vi "CSM DQMH-Style Template.vi"(7 "Name (\"\" to Use UUID)":string="CSM-Module") -> ()   [LabVIEW 2017]
doc: "------------- lvcsm -------------\n[CSMStates]\nItem 0 = \"Idle\"\nItem 1 = \"CSM Documentation\"\nItem 2 = \"VI Reference\"\nItem 3 = \"Error Handler\"\nItem 4 = \"Critical Error\"\nItem 5 = \"Target Timeout Error\"\nItem 6 = \"Target Error\"\nItem 7 = \"Async Response\"\nItem 8 = \"Response\"\nItem 9 = \"Async Message Posted\"\nItem 10 = \"Initialize Core Data\"\nItem 11 = \"Exit\"\nItem 12 = \"Data: Initialize\"\nItem 13 = \"Data: Update Indicators\"\nItem 14 = \"Data: Cleanup\"\nItem 15 = \"Macro: Initialize\"\nItem 16 = \"Macro: Exit\"\nItem 17 = \"API: API1\"\nItem 18 = \"API: API2\"\nItem 19 = \"Action: action1\"\nItem 20 = \"Action: action2\"\n\n[CSMStatus]\nItem 0 = \"Error Occurred@Error Handler\""
uses:
  user.lib/_NEVSTOP/Communicable State Machine(CSM)/AdvanceAPI/CSM - Revert Arguments-Safe String.vi
  user.lib/_NEVSTOP/Communicable State Machine(CSM)/AdvanceAPI/CSM - Break Down Multiple States String.vi
  user.lib/_NEVSTOP/Communicable State Machine(CSM)/AdvanceAPI/CSM - Compact Multiple States.vi
  user.lib/_NEVSTOP/Communicable State Machine(CSM)/AdvanceAPI/CSM - Make String Arguments Safe.vi
  user.lib/_NEVSTOP/Communicable State Machine(CSM)/AdvanceAPI/CSM - Keywords.vi
  user.lib/_NEVSTOP/Communicable State Machine(CSM)/_Shared/Trim Single-line Text.vi
  user.lib/_NEVSTOP/Communicable State Machine(CSM)/_Polymophic/CSM - Filter Duplicated Lines.vi
  user.lib/_NEVSTOP/Communicable State Machine(CSM)/Communicable State Machine.lvlib
panel:
  in  "Slide":dbl(slide) caption="Flood of Events:\n\nPanel/Pane Size Event\nSlide/Knob... User Event by dragging\nNumeric Control Value Change Event by Arraw Button" scale=0.0..10.0
  out "Error Occurred":errorcluster
  out "State History":string
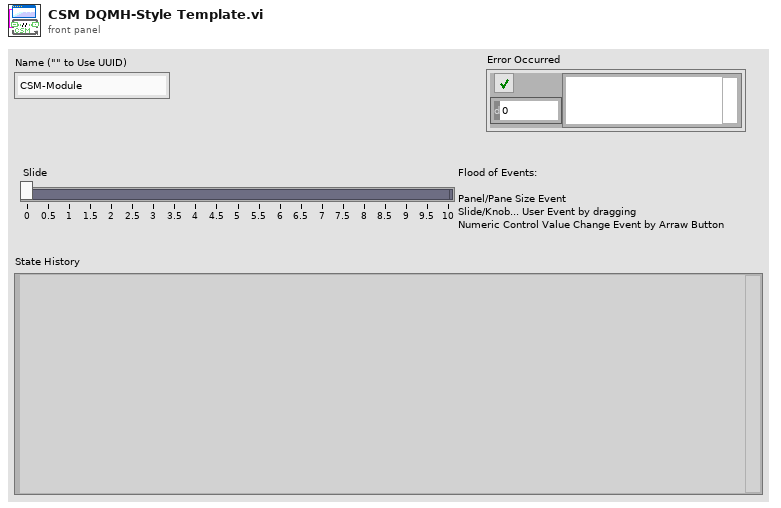
[diagram p1: front panel]
types:
  T1 = enum32{"Invalid", "Standard", "Closed", "Hidden", "Minimized", "Maximized"}
  T2 = enum32{"invalid app kind", "Development System", "Run Time System", "Student Edition", "Embedded LabVIEW", "Evaluation", "Custom"}
  T3 = typedef "Communicable State Machine.lvlib/_CSM_Response Source Message.ctl" = cluster{"‘State":string, "’Arguments":string, "’Error":errorcluster}
  T4 = cluster{"Current VI Reference":refnum<vi>, "Close Panel on Exit?":bool}
  T5 = cluster{"Core":cluster{"Current VI Reference":refnum<vi>, "Close Panel on Exit?":bool}, "Your Boolean data":bool, "Your string data":string}
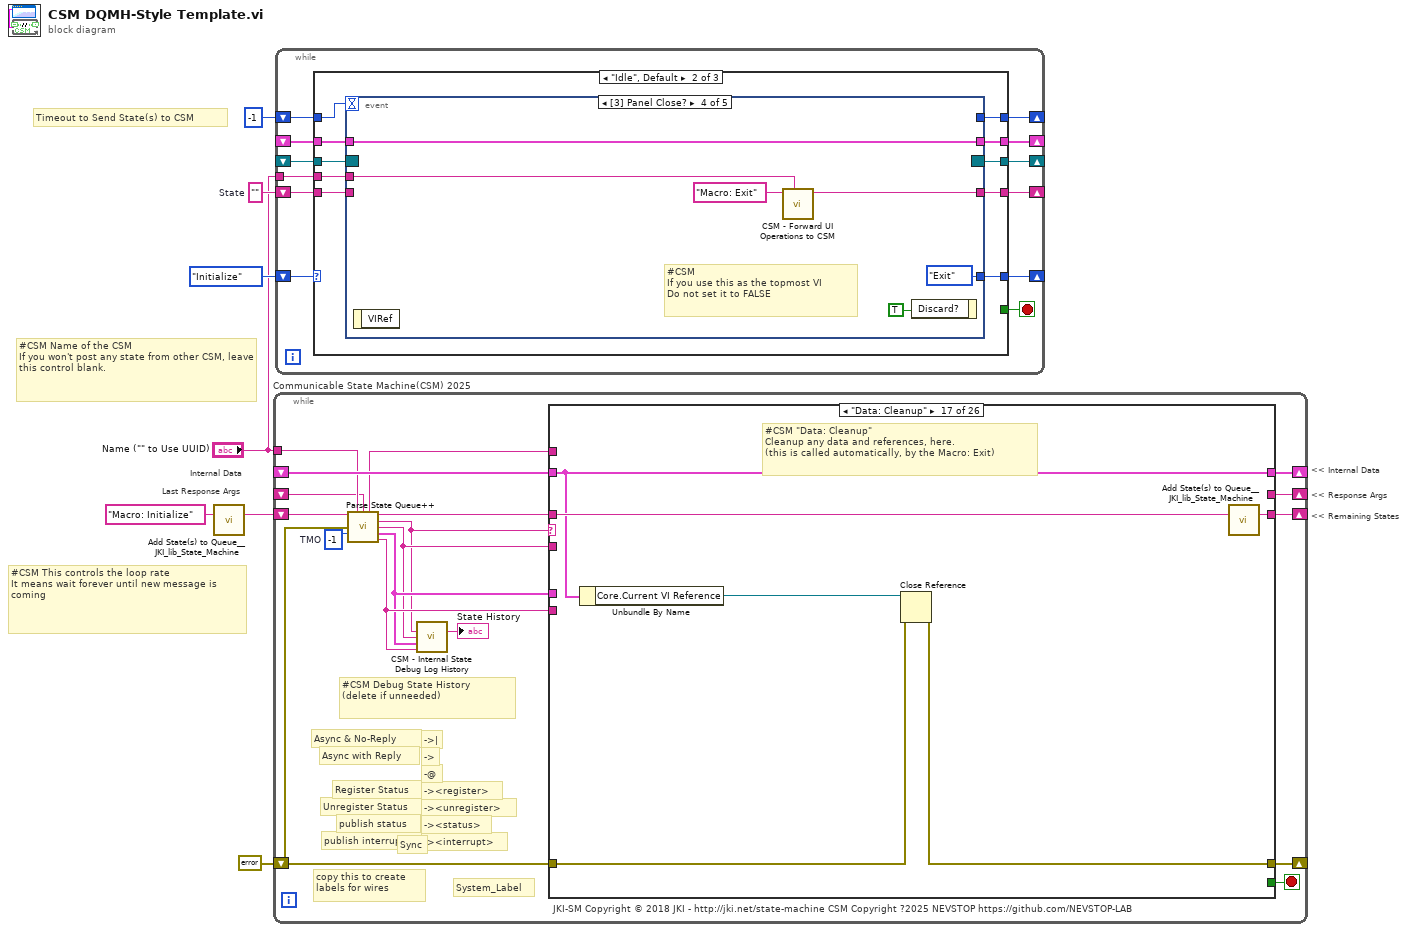
[diagram p0: block diagram]
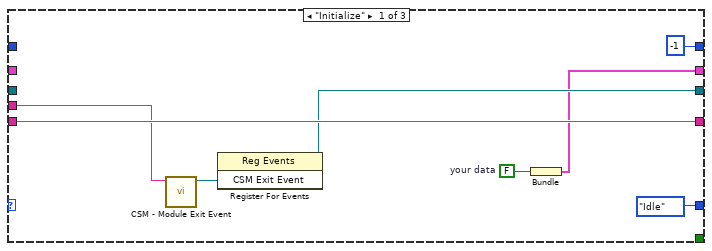
[diagram p2: hidden frame]
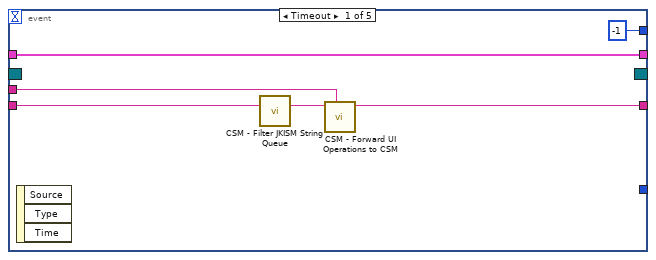
[diagram p3: hidden frame]
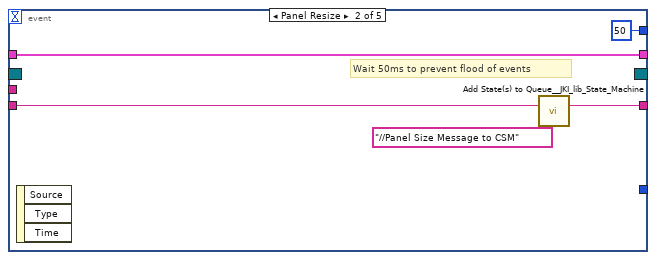
[diagram p4: hidden frame]
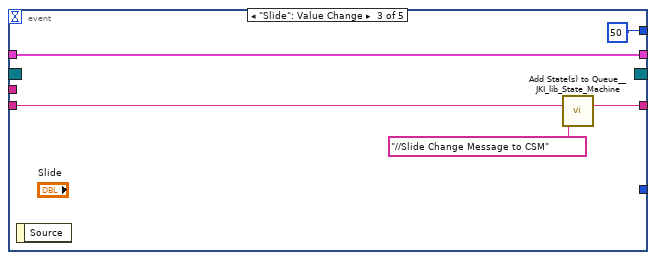
[diagram p5: hidden frame]
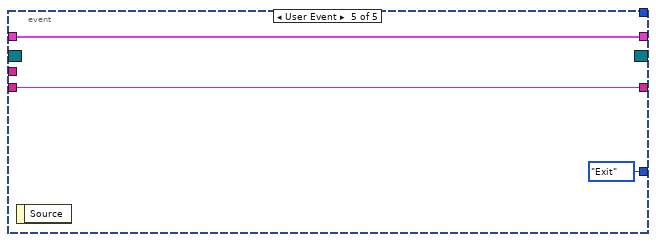
[diagram p6: hidden frame]
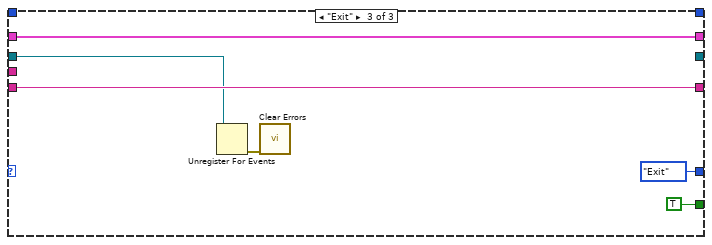
[diagram p7: hidden frame]
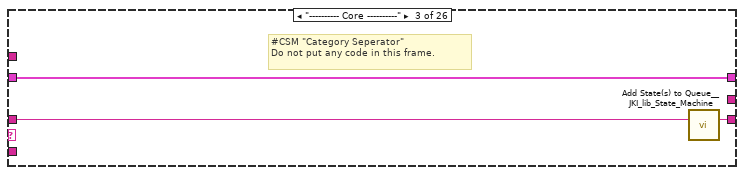
[diagram p10: hidden frame]
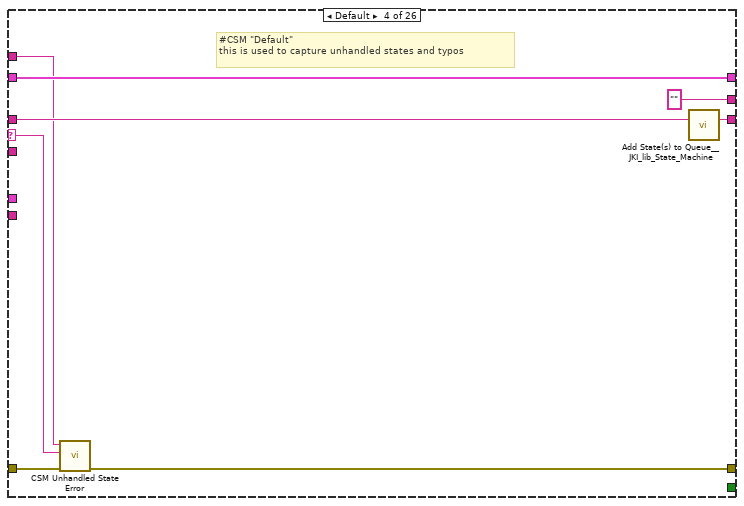
[diagram p11: hidden frame]
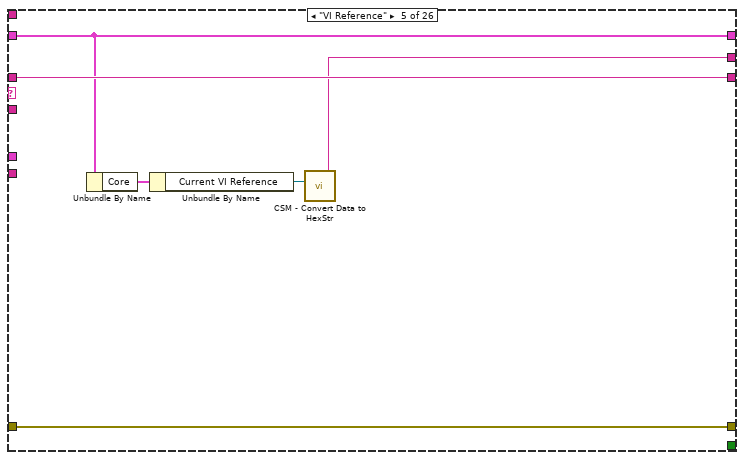
[diagram p12: hidden frame]
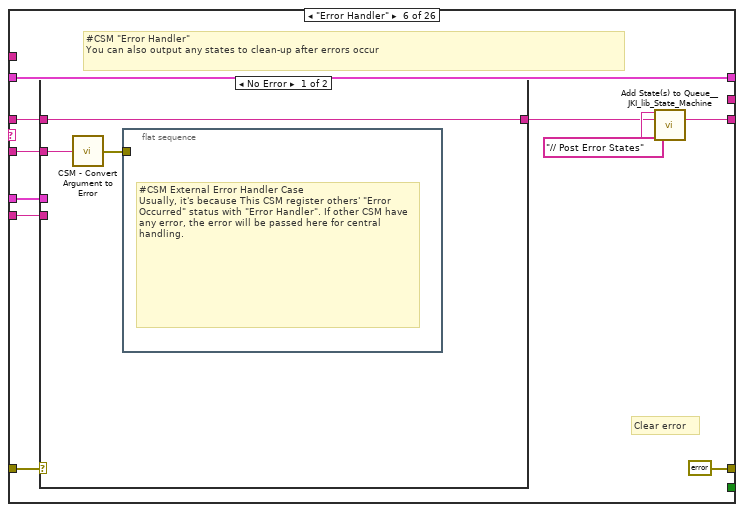
[diagram p13: hidden frame]
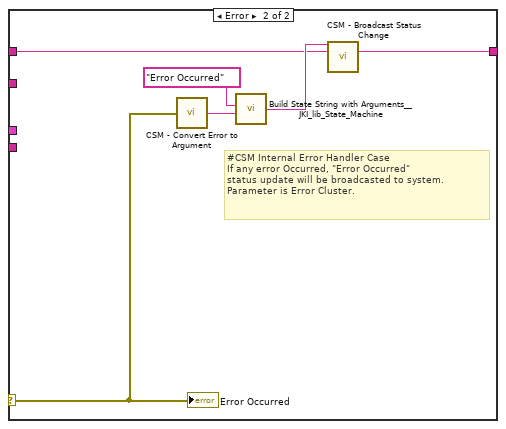
[diagram p14: hidden frame]
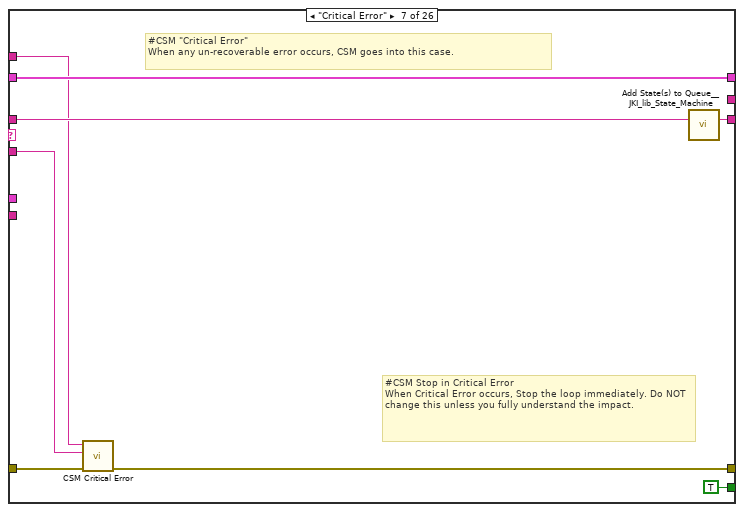
[diagram p15: hidden frame]
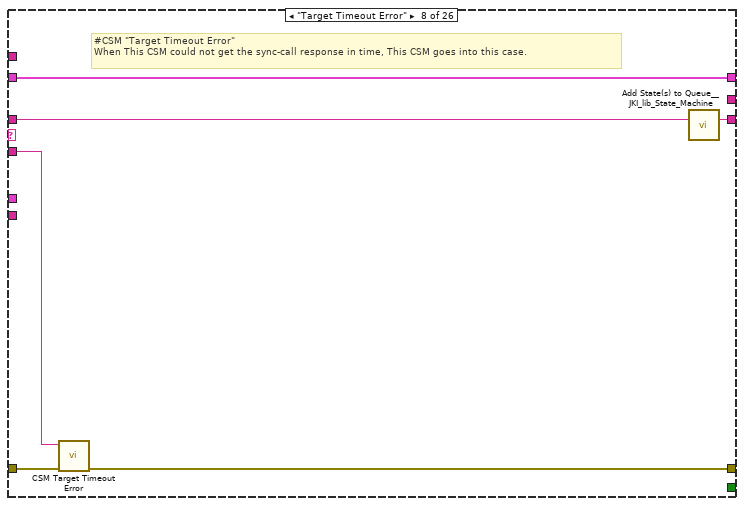
[diagram p16: hidden frame]
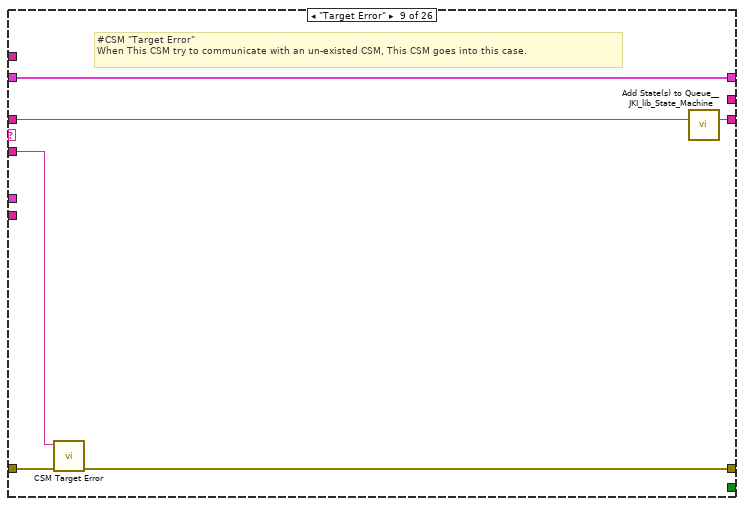
[diagram p17: hidden frame]
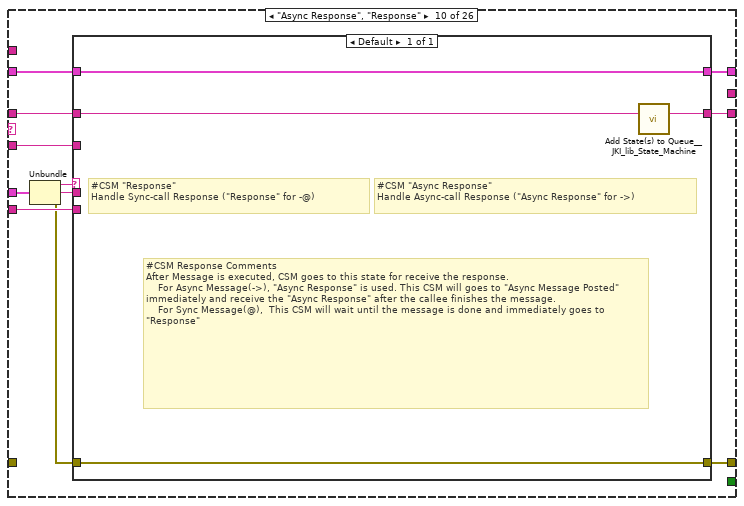
[diagram p18: hidden frame]
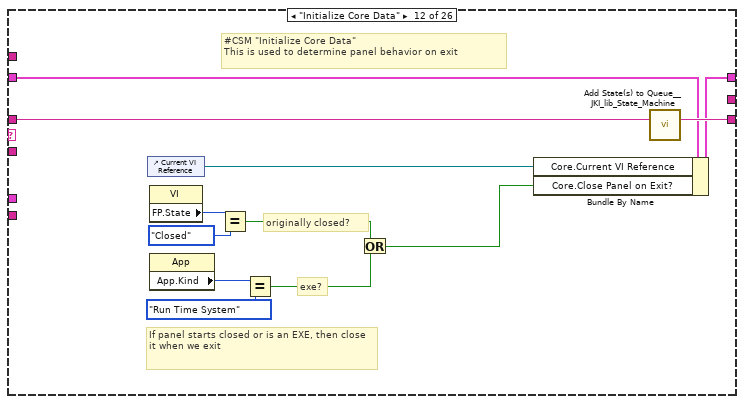
[diagram p20: hidden frame]
diagram:
  w3 = ""  # State
  # "Timeout to Send State(s) to CSM"
  # "Last Response Args"
  # "Internal Data"
  # "#CSM Name of the CSM\nIf you won't post any state from other CSM, leave this control blank."
  # "#CSM This controls the loop rate\nIt means wait forever until new message is coming"
  # "<< Internal Data"
  # "<< Response Args"
  # "<< Remaining States"
  n1 = call <vilib>:"Add State(s) to Queue__JKI_lib_State_Machine.vi"("State(s) in (\"\")"="Macro: Initialize" ("Init State(\"Macro: Initialize\")")) -> ("States Out"=w7:string)  [unwired: 14 in]
  n2 = while "Communicable State Machine(CSM) 2025" {
    shift-right: [w20] -> _
    shift-left: _ -> [w19]
    shift-right: [w23] -> _
    shift-left: errorcluster {"status"=FALSE, "code"=0, "source"=""} ("error out") -> [w9]
    shift-right: [w22] -> _
    shift-left: w7 -> [w24]
    tunnel: "Name (\"\" to Use UUID)" -> [w16]
    shift-right: [w17] -> _
    shift-left: _ -> [w11]
    stop <- w21 stop-if-true
    w18 = -1  # TMO
    # "#CSM Debug State History\n(delete if unneeded)"
    # "-><interrupt>"
    # "-><status>"
    # "-><unregister>"
    # "-><register>"
    # "-@"
    # "->"
    # "->|"
    # "publish interrupt"
    # "publish status"
    # "Unregister Status"
    # "Register Status"
    # "Sync"
    # "Async with Reply"
    # "Async & No-Reply"
    # "JKI-SM Copyright © 2018 JKI - http://jki.net/state-machine CSM Copyright ?2025 NEVSTOP https://github.com/NEVSTOP-LAB"
    # "copy this to create labels for wires"
    # "System_Label"
    n3 = call "Parse State Queue++.vi"("State Queue"=w24, "Name (\"\" to Use UUID)"=w16, "Response Arguments"=w11, "Previous Error"=w9, "Dequeue (1 ms)"=w18) -> ("Name Used"=w10:string, "Remaining States"=w25:string, "Current State"=w12:string, "Arguments"=w13:string, "Additional Information"=w14:T3, "Source CSM"=w15:string)  [unwired: 5 in]
    n4 = call "CSM - Internal State Debug Log History.vi"("State"=w12, "Arguments (\"\")"=w13, ">> Response Source Message >>"=w14, "Source (\"\")"=w15) -> ("Debug Log"=→"State History":string)  [unwired: 11 in]
    n5 = case shown="\"Data: Cleanup\"" w12 {
      selector: w12 -> [_ _ _ w36 _ _ _ _ _ _ _ _ _ _ _ _ _ _ _ _ _ _ _ _ _ _]
      tunnel: w25 -> [w26 w29 w32 w40 w45 w50 w73 w79 w85 w95 w102 w114 w118 w121 w127 w129 w135 w138 w142 w148 w150 w153 w157 w162 w165 w168]
      tunnel: w13 -> [_ _ _ _ _ w49 w69 w76 w82 w89 _ _ _ _ _ _ _ _ _ _ _ _ w155 _ _ _]
      tunnel: w19 -> [w27 w28 w30 w38 w44 w55 w71 w77 w83 w93 w101 w108 w116 w119 _ w128 w130 w136 w140 w146 w149 w152 w156 w160 w163 w166]
      tunnel: [_ _ _ w33 w46 errorcluster {"status"=FALSE, "code"=0, "source"=""} ("error out") w66 w74 w80 w96 _ _ _ _ _ _ w131 _ _ _ _ _ _ _ _ _] -> w23
      tunnel: w9 -> [_ _ _ w34 w46 w53 w67 w75 w81 _ _ _ _ _ _ _ w132 _ _ _ _ _ _ _ _ _]
      tunnel: [w26 w29 w31 w39 w45 w51 w72 w78 w84 w94 w102 w113 w117 w120 w126 w129 w134 w137 w141 w147 w150 w153 w157 w161 w164 w167] -> w22
      tunnel: [_ _ _ _ _ _ TRUE _ _ _ _ _ TRUE _ _ _ _ _ _ _ _ _ _ _ _ _] -> w21
      tunnel: [w27 w28 w30 w38 w44 w55 w71 w77 w83 w92 w101 w112 w116 w119 w125 w128 w130 w136 w140 w146 w149 w152 w156 w160 w163 w166] -> w20
      tunnel: w15 -> [_ _ _ _ _ w48 _ _ _ w90 _ _ _ _ _ _ _ _ _ _ _ _ _ _ _ _]
      tunnel: w14 -> [_ _ _ _ _ w47 _ _ _ w91 _ _ _ _ _ _ _ _ _ _ _ _ _ _ _ _]
      tunnel: [_ _ _ "" w41 _ _ _ _ _ _ _ _ _ _ _ _ _ _ _ _ "API1 Response" w154 _ _ _] -> w17
      tunnel: w10 -> [_ _ _ w35 _ _ w68 _ _ _ _ _ _ _ _ _ _ _ _ _ _ _ _ _ _ _]
      frame "", "Idle" {
        # "#CSM \"Idle/Event Handler\"\nexecutes when the state queue is empty"
      }
      frame "CSM Documentation" {
        # "#CSM State Syntax\n\n// Comment line, all text to the right of “//” will be ignored\n// Local Message Example\nDoSth: DoA >> Arguments\n\n// Sync Call Example\nAPI: xxxx >> Arguments -@ TargetModule\n\n// Async Call Example\nAPI: xxxx >> Arguments -> TargetModule\n\n// Async Call without Reply Example\nAPI: xxxx >> Arguments ->| TargetModule\n\n// Broadcast normal status:\nStatus >> StatusArguments  -><status>\n\n// Broadcast Interrupt status:\nInterrupt >> StatusArguments  -><interrupt>\n\n// Register Source Module's status to Handler Module\nStatus@Source Module >> Handler Module@Handler Module -><register>\n\n// Unegister Source Module's status\nStatus@Source Module >> Handler Module -><unregister>"
        # "#CSM README FIRST\n\nCommunicable State Machine(CSM) is a LabVIEW application framework that builds upon JKI State Machine(JKISM). It follows the pattern of JKISM and extends the keywords to describe message communication between modules, including concepts such as Sync-Message, Async-Message, Subscription/Unsubscription of status - essential elements for creating reusable code modules. For more information, please visit the CSM wiki: https://nevstop-lab.github.io/CSM-Wiki/\n\nFor instructions on JKI State Machine, visit: \n    http://jki.net/state-machine/\nFor information about CSM, visit: \n    https://github.com/NEVSTOP-LAB"
        # "#CSM \"Documentation\"\nCase for holding CSM Documenation"
      }
      frame "---------- Core ----------" {
        # "#CSM \"Category Seperator\"\nDo not put any code in this frame."
        n6 = call <vilib>:"Add State(s) to Queue__JKI_lib_State_Machine.vi"("State(s) in (\"\")"=w32) -> ("States Out"=w31:string)  [unwired: 14 in]
      }
      frame Default {
        # "#CSM \"Default\"\nthis is used to capture unhandled states and typos"
        n7 = call "CSM Unhandled State Error.vi"("error in (no error)"=w34, "Undefined State"=w36, "CSM Name"=w35) -> ("error out"=w33:errorcluster)  [unwired: 8 in]
        n8 = call <vilib>:"Add State(s) to Queue__JKI_lib_State_Machine.vi"("State(s) in (\"\")"=w40) -> ("States Out"=w39:string)  [unwired: 14 in]
      }
      frame "VI Reference" {
        n9 = Unbundle By Name(w44) -> ("Core"=w43:T4)
        n10 = Unbundle By Name(w43) -> ("Current VI Reference"=w42:refnum<vi>)
        n11 = call "CSM - Convert Data to HexStr.vi"("Variant"=w42) -> ("HEX String (0-9,A-F)"=w41:string)  [unwired: 8 in]
      }
      frame "Error Handler" {
        # "#CSM \"Error Handler\"\nYou can also output any states to clean-up after errors occur"
        # "Clear error"
        n12 = case shown="No Error" w53 {
          selector: w53 -> [_ w60]
          tunnel: [w59 w62] -> w52
          tunnel: w50 -> [w59 w61]
          tunnel: w49 -> [w58 _]
          tunnel: w48 -> [_ _]
          tunnel: w47 -> [_ _]
          frame No Error {
            n13 = call "CSM - Convert Argument to Error.vi"("Argument"=w58) -> ("Error"=w57:errorcluster)  [unwired: 4 in]
            n14 = flat-sequence {
              tunnel: w57 -> [_]
              frame #0 {
                # "#CSM External Error Handler Case\nUsually, it's because This CSM register others' \"Error Occurred\" status with \"Error Handler\". If other CSM have any error, the error will be passed here for central handling."
              }
            }
          }
          frame Error {
            # "#CSM Internal Error Handler Case \nIf any error Occurred, \"Error Occurred\" \nstatus update will be broadcasted to system.\nParameter is Error Cluster."
            n15 = call "CSM - Convert Error to Argument.vi"("Error"=w60) -> ("Argument"=w64:string)  [unwired: 4 in]
            n16 = call <vilib>:"Build State String with Arguments__JKI_lib_State_Machine.vi"("Arguments (\"\")"=w64, "State"="Error Occurred" ("Status with Arguments")) -> ("State with Arguments"=w63:string)  [unwired: 4 in]
            n17 = call "CSM - Broadcast Status Change.vi"("Status With Arguments"=w63, "State Queue"=w61) -> ("Remaining States"=w62:string)  [unwired: 13 in]
            "Error Occurred" <- w60
          }
        }
        n18 = call <vilib>:"Add State(s) to Queue__JKI_lib_State_Machine.vi"("State(s) in Front (\"\")"="// Post Error States", "State(s) in (\"\")"=w52) -> ("States Out"=w51:string)  [unwired: 13 in]
      }
      frame "Critical Error" {
        # "#CSM \"Critical Error\"\nWhen any un-recoverable error occurs, CSM goes into this case."
        # "#CSM Stop in Critical Error\nWhen Critical Error occurs, Stop the loop immediately. Do NOT change this unless you fully understand the impact."
        n19 = call "CSM Critical Error.vi"("error in (no error)"=w67, "Arugments (As Reason)"=w69, "CSM Name"=w68) -> ("error out"=w66:errorcluster)  [unwired: 8 in]
        n20 = call <vilib>:"Add State(s) to Queue__JKI_lib_State_Machine.vi"("State(s) in (\"\")"=w73) -> ("States Out"=w72:string)  [unwired: 14 in]
      }
      frame "Target Timeout Error" {
        # "#CSM \"Target Timeout Error\"\nWhen This CSM could not get the sync-call response in time, This CSM goes into this case."
        n21 = call "CSM Target Timeout Error.vi"("error in (no error)"=w75, "Arguments (As CSM Name)"=w76) -> ("error out"=w74:errorcluster)  [unwired: 9 in]
        n22 = call <vilib>:"Add State(s) to Queue__JKI_lib_State_Machine.vi"("State(s) in (\"\")"=w79) -> ("States Out"=w78:string)  [unwired: 14 in]
      }
      frame "Target Error" {
        # "#CSM \"Target Error\"\nWhen This CSM try to communicate with an un-existed CSM, This CSM goes into this case."
        n23 = call "CSM Target Error.vi"("error in (no error)"=w81, "Arguments (As CSM Name)"=w82) -> ("error out"=w80:errorcluster)  [unwired: 9 in]
        n24 = call <vilib>:"Add State(s) to Queue__JKI_lib_State_Machine.vi"("State(s) in (\"\")"=w85) -> ("States Out"=w84:string)  [unwired: 14 in]
      }
      frame "Async Response", "Response" {
        n25 = Unbundle(w91) -> ("‘State"=w88:string, "’Arguments"=w87:string, "’Error"=w86:errorcluster)
        n26 = case shown="Default" w88 {
          tunnel: [w97] -> w94
          tunnel: w95 -> [w98]
          tunnel: [w100] -> w92
          tunnel: w93 -> [w100]
          tunnel: [w99] -> w96
          tunnel: w86 -> [w99]
          tunnel: w90 -> [_]
          tunnel: w89 -> [_]
          tunnel: w87 -> [_]
          frame Default {
            # "#CSM \"Async Response\"\nHandle Async-call Response (\"Async Response\" for ->)"
            # "#CSM \"Response\"\nHandle Sync-call Response (\"Response\" for -@)"
            # "#CSM Response Comments\nAfter Message is executed, CSM goes to this state for receive the response.\n    For Async Message(->), \"Async Response\" is used. This CSM will goes to \"Async Message Posted\" immediately and receive the \"Async Response\" after the callee finishes the message.\n    For Sync Message(@),  This CSM will wait until the message is done and immediately goes to \"Response\""
            n27 = call <vilib>:"Add State(s) to Queue__JKI_lib_State_Machine.vi"("State(s) in (\"\")"=w98) -> ("States Out"=w97:string)  [unwired: 14 in]
          }
        }
      }
      frame "Async Message Posted" {
        # "#CSM \"Async Message Posted\"\nAfter Async Message is posted (-> or ->| ), CSM goes to this state for post-action.\nYou can use Argument - State to tell which Async Message is called."
      }
      frame "Initialize Core Data" {
        # "#CSM \"Initialize Core Data\"\nThis is used to determine panel behavior on exit"
        # "originally closed?"
        # "exe?"
        # "If panel starts closed or is an EXE, then close it when we exit"
        n28 = control-ref of="Current VI Reference"() -> (w106:refnum<vi>)
        n29 = property class="VI"() -> ("FP.State"=w105:T1)  [unwired: 2 in, 2 out]
        n30 = property class="App"() -> ("App.Kind"=w111:T2)  [unwired: 2 in, 2 out]
        n31 = Equal?(x=w105, y=T1."Closed" ("Front Panel Window:State")) -> (x = y?=w103:bool)
        n32 = Equal?(x=w111, y=T2."Run Time System" ("Application:Kind")) -> (x = y?=w109:bool)
        n33 = Or(x=w103, y=w109) -> (x .or. y?=w107:bool)
        n34 = Bundle By Name(cluster=w108, "Core.Current VI Reference"=w106, "Core.Close Panel on Exit?"=w107) -> (w112:T5)
        n35 = call <vilib>:"Add State(s) to Queue__JKI_lib_State_Machine.vi"("State(s) in (\"\")"=w114) -> ("States Out"=w113:string)  [unwired: 14 in]
      }
      frame "Exit" {
        # "#CSM \"Exit\"\nCase for exiting the loop. No errors that occur here will be handled."
        n36 = call <vilib>:"Add State(s) to Queue__JKI_lib_State_Machine.vi"("State(s) in (\"\")"=w118) -> ("States Out"=w117:string)  [unwired: 14 in]
      }
      frame "---------- Data ----------" {
        # "#CSM \"Category Seperator\"\nDo not put any code in this frame."
        n37 = call <vilib>:"Add State(s) to Queue__JKI_lib_State_Machine.vi"("State(s) in (\"\")"=w121) -> ("States Out"=w120:string)  [unwired: 14 in]
      }
      frame "Data: Initialize" {
        w122 = T4 {"Current VI Reference"=refnum, "Close Panel on Exit?"=FALSE}  # Core
        w124 = TRUE  # Your Boolean data
        w123 = ""  # Your string data
        # "#CSM \"Data: Initialize\"\nInitialize the shift-register data, here.\n(data names are defined by what you wire into the bundle function)"
        # "#CSM do not delete - used by framework"
        # "#CSM Expand Bundle to add new data elements to shift register data."
        # "#CSM Add new data here."
        # "#CSM Data names and types of shift register data are defined by this bundle."
        n38 = Bundle("Core"=w122, "Your Boolean data"=w124, "Your string data"=w123) -> (w125:T5)  [unwired: 1 in]
        n39 = call <vilib>:"Add State(s) to Queue__JKI_lib_State_Machine.vi"("State(s) in (\"\")"=w127) -> ("States Out"=w126:string)  [unwired: 14 in]
      }
      frame "Data: Update Indicators" {
      }
      frame "Data: Cleanup" {
        # "#CSM \"Data: Cleanup\"\nCleanup any data and references, here.\n(this is called automatically, by the Macro: Exit)"
        n40 = Unbundle By Name(w130) -> ("Core.Current VI Reference"=w133:refnum<vi>)
        n41 = Close Reference(reference=w133, error in (no error)=w132) -> (error out=w131:errorcluster)
        n42 = call <vilib>:"Add State(s) to Queue__JKI_lib_State_Machine.vi"("State(s) in (\"\")"=w135) -> ("States Out"=w134:string)  [unwired: 14 in]
      }
      frame "---------- Macro ----------" {
        # "#CSM \"Category Seperator\"\nDo not put any code in this frame."
        n43 = call <vilib>:"Add State(s) to Queue__JKI_lib_State_Machine.vi"("State(s) in (\"\")"=w138) -> ("States Out"=w137:string)  [unwired: 14 in]
      }
      frame "Macro: Initialize" {
        # "#CSM \"Macro: Initialize\"\nInitialization Macro (This is called once, when the VI starts)"
        n44 = call <vilib>:"Add State(s) to Queue__JKI_lib_State_Machine.vi"("State(s) in Front (\"\")"="Data: Initialize\nInitialize Core Data\nData: Update Indicators", "State(s) in (\"\")"=w142) -> ("States Out"=w141:string)  [unwired: 13 in]
      }
      frame "Macro: Exit" {
        # "#CSM \"Macro: Exit\"\nExit Macro (This is called once, when the VI exits)"
        n45 = call <vilib>:"Add State(s) to Queue__JKI_lib_State_Machine.vi"("State(s) in Front (\"\")"="//Exit Sub-Modules ", "State(s) at Back (\"\")"="Data: Cleanup\nExit") -> ("States Out"=w144:string)  [unwired: 13 in]
        n46 = call <vilib>:"Add State(s) to Queue__JKI_lib_State_Machine.vi"("State(s) in Front (\"\")"=w144, "State(s) in (\"\")"=w148) -> ("States Out"=w147:string)  [unwired: 13 in]
      }
      frame "---------- API ----------" {
        # "#CSM \"Category Seperator\"\nDo not put any code in this frame."
      }
      frame "API: API1" {
        # "#CSM API Example\nCopy/Rename this case for your own API"
        # "#CSM >> Source CSM >>\nIf you need to tell who triggered this state , use this string. If it's this case itself, this string is \"\"."
        # "#CSM >> Arguments >>\nDeal with the parameter if any"
        # "#CSM Response\nConnect this to return the response of your API"
      }
      frame "API: API2" {
        # "#CSM API Example\nCopy/Rename this case for your own API"
        # "unpack Hex String  to Variant\nif complex parameter is needed."
        n47 = call "CSM - Convert HexStr to Data.vi"("HEX String"=w155) -> ()  [unwired: 7 in, 2 out]
        n48 = disable-structure shown="Disabled" {
          disable-tunnel: [w158 "API2 Response"] -> w154
          frame Disabled {
            # "pack variant to hexstr \nif complex response is needed."
            # "complex Response"
            n49 = call "CSM - Convert Data to HexStr.vi"() -> ("HEX String (0-9,A-F)"=w158:string)  [unwired: 9 in]
          }
          frame Enabled {
          }
        }
      }
      frame "---------- Action ----------" {
        # "#CSM \"Category Seperator\"\nDo not put any code in this frame."
        n50 = call <vilib>:"Add State(s) to Queue__JKI_lib_State_Machine.vi"("State(s) in (\"\")"=w162) -> ("States Out"=w161:string)  [unwired: 14 in]
      }
      frame "Action: action1" {
        # "#CSM \"Internal State\"\nThis category is used for holding internal states"
        n51 = call <vilib>:"Add State(s) to Queue__JKI_lib_State_Machine.vi"("State(s) in (\"\")"=w165) -> ("States Out"=w164:string)  [unwired: 14 in]
      }
      frame "Action: action2" {
        # "#CSM \"Internal State\"\nThis category is used for holding internal states"
        n52 = call <vilib>:"Add State(s) to Queue__JKI_lib_State_Machine.vi"("State(s) in (\"\")"=w168) -> ("States Out"=w167:string)  [unwired: 14 in]
      }
    }
  }
  n53 = while {
    shift-right: [w179] -> _
    shift-left: enum16{"Idle", "Initialize", "Exit"}."Initialize" -> [w180]
    tunnel: "Name (\"\" to Use UUID)" -> [w177]
    shift-right: [w175] -> _
    shift-left: w3 -> [w176]
    shift-right: [w173] -> _
    shift-left: -1 -> [w174]
    shift-right: [w172] -> _
    shift-left: _ -> [w171]
    shift-right: [w170] -> _
    shift-left: _ -> [w169]
    stop <- w178 stop-if-true
    n54 = case shown="\"Idle\", Default" w180 {
      tunnel: [enum16{"Idle", "Initialize", "Exit"}."Idle" w198 enum16{"Idle", "Initialize", "Exit"}."Exit"] -> w179
      tunnel: [_ _ TRUE] -> w178
      tunnel: w177 -> [w184 w197 _]
      tunnel: w176 -> [w187 w195 w227]
      tunnel: [w187 w196 w227] -> w175
      tunnel: w174 -> [_ w193 _]
      tunnel: [-1 w194 _] -> w173
      tunnel: [w183 w191 _] -> w172
      tunnel: w171 -> [_ w192 w226]
      tunnel: [w181 w189 w224] -> w170
      tunnel: w169 -> [_ w190 w224]
      frame "Initialize" {
        w182 = FALSE  # your data
        n55 = call "CSM - Module Exit Event.vi"("Name (\"\" to Use UUID) In"=w184) -> ("CSM Exit Event"=w185:refnum<user-event>)  [unwired: 8 in, 2 out]
        n56 = register-events(w185) -> (reference out=w183:refnum<event-registration>)  [unwired: 2 in, 1 out]
        n57 = Bundle("your data"=w182) -> (w181:cluster{"your data":bool})  [unwired: 1 in]
      }
      frame "Idle", Default {
        n58 = event shown="[3] Panel Close?" {
          selector: w192 -> [_ _ _ _ _]
          dyn-events: [_ _ _ _ _] -> w191
          timeout: w193 -> [_ _ _ _ _]
          tunnel: [_ _ _ enum16{"Idle", "Initialize", "Exit"}."Exit" enum16{"Idle", "Initialize", "Exit"}."Exit"] -> w198
          tunnel: w197 -> [w200 _ _ w217 _]
          tunnel: w195 -> [w203 w209 w214 _ w223]
          tunnel: [w201 w208 w213 w216 w223] -> w196
          tunnel: [-1 50 50 _ _] -> w194
          tunnel: w190 -> [w199 w205 w210 w215 w221]
          tunnel: [w199 w205 w210 w215 w221] -> w189
          event Timeout {
            n59 = event-data() -> ()  [unwired: 1 in, 3 out]
            n60 = call-poly "CSM - Filter JKISM String Queue.vi"("States In"=w203) -> ("States Out"=w202:string)  [unwired: 14 in]
            n61 = call "CSM - Forward UI Operations to CSM.vi"("Name (\"\" to Use UUID)"=w200, "State (S) In (\"\")"=w202) -> ("States Out"=w201:string)  [unwired: 9 in]
          }
          event Panel Resize {
            # "Wait 50ms to prevent flood of events"
            n62 = event-data() -> ()  [unwired: 1 in, 3 out]
            n63 = call <vilib>:"Add State(s) to Queue__JKI_lib_State_Machine.vi"("State(s) in (\"\")"=w209, "State(s) at Back (\"\")"="//Panel Size Message to CSM" ("State(s) at Back (\"\")")) -> ("States Out"=w208:string)  [unwired: 13 in]
          }
          event "Slide": Value Change {
            n64 = event-data() -> ()  [unwired: 1 in, 1 out]
            n65 = call <vilib>:"Add State(s) to Queue__JKI_lib_State_Machine.vi"("State(s) in (\"\")"=w214, "State(s) at Back (\"\")"="//Slide Change Message to CSM" ("State(s) at Back (\"\")")) -> ("States Out"=w213:string)  [unwired: 13 in]
          }
          event Panel Close? {
            # "#CSM \nIf you use this as the topmost VI\nDo not set it to FALSE"
            n66 = event-data() -> ()  [unwired: 1 in, 1 out]
            n67 = call "CSM - Forward UI Operations to CSM.vi"("Name (\"\" to Use UUID)"=w217, "State (S) In (\"\")"="Macro: Exit" ("State")) -> ("States Out"=w216:string)  [unwired: 9 in]
            n68 = event-data("Discard?"=TRUE) -> ()  [unwired: 1 in, 1 out]
          }
          event User Event {
            n69 = event-data() -> ()  [unwired: 1 in, 1 out]
          }
        }
      }
      frame "Exit" {
        n70 = Unregister For Events(event registration refnum=w226) -> (error out=w225:errorcluster)  [unwired: 1 in]
        n71 = call <vilib>:"Clear Errors.vi"("error in (no error)"=w225) -> ()  [unwired: 5 in, 2 out]
      }
    }
  }
